vi "CANbus Wrapper.vi"(0 "Signals IN":T4[](array[typedef])=[{"XNET Signal"="GIP_TestModeFlag\nDatabase", "Data"=0.0}, {"XNET Signal"="StatusLED\nDatabase", "Data"=0.0}, {"XNET Signal"="FaultLED\nDatabase", "Data"=0.0}, {"XNET Signal"="Relay\nDatabase", "Data"=0.0}, {"XNET Signal"="ESP32Comms\nDatabase", "Data"=0.0}], 1 "Method":T5=enum."Write Sigs Session", 2 "JSON signals file":path, 3 "DBC File":path, 5 "Frames IN":T1[](array[typedef]) {"Raw Frame"."payload" format="%x"; "Raw Frame"."timestamp" format="%<%.7X\n%x>T"; "Raw Frame"."type" items=["CAN Data"=0, "CAN Remote"=1, "CAN Bus Error"=2, "CAN 2.0 Data"=8, "CAN FD Data"=16, "CAN FD+BRS Data"=24, "J1939 Data"=192, "Delay"=224, "Log Trigger"=225, "Start Trigger"=226]; "Raw Frame"."identifier" format="%x"}, 7 "Baud Rate":u64=1000000, 9 "Termination":u32(ring) items=["Off", "On"], 11 "error in (no error)":errorcluster, 12 "interface":refnum<k21>="CAN2") -> (4 "Signals OUT":T4[](array[typedef]), 6 "Frames OUT":T1[](array[typedef]) {"Raw Frame"."payload" format="%x"; "Raw Frame"."timestamp" format="%<%.7X\n%x>T"; "Raw Frame"."type" items=["CAN Data"=0, "CAN Remote"=1, "CAN Bus Error"=2, "CAN 2.0 Data"=8, "CAN FD Data"=16, "CAN FD+BRS Data"=24, "J1939 Data"=192, "Delay"=224, "Log Trigger"=225, "Start Trigger"=226]; "Raw Frame"."identifier" format="%x"}, 15 "error out":errorcluster)   [LabVIEW 2021]
uses:
  controls/BCS Manager.ctl
  controls/Signal Data.ctl
  controls/Frame Data.ctl
  <vilib>/xnet/xnet.llb/XNET Frame CAN.ctl
  <vilib>/xnet/xnet.llb/XNET Frame Type CAN.ctl
  controls/Signal Tracker.ctl
  <vilib>/xnet/xnet.llb/XNET Create Session (Frame Input Single-point).vi
  <vilib>/xnet/xnet.llb/XNET Create Session (Frame Output Single-point).vi
  <vilib>/xnet/xnet.llb/XNET Create Session (Signal Input Single-point).vi
  <vilib>/xnet/xnet.llb/XNET Create Session (Signal Output Single-point).vi
  <vilib>/xnet/xnet.llb/XNET Write (Signal Single-point).vi
  <vilib>/xnet/xnet.llb/XNET Create Session (Conversion).vi
  <vilib>/xnet/xnet.llb/XNET Convert (Signal to Frame CAN).vi
  <vilib>/xnet/xnet.llb/XNET Write (Frame CAN).vi
  <vilib>/xnet/xnet.llb/XNET Read (Signal Single-point).vi
  <vilib>/xnet/xnet.llb/XNET Read (Frame CAN).vi
  <resource>/objmgr/xnet.rc
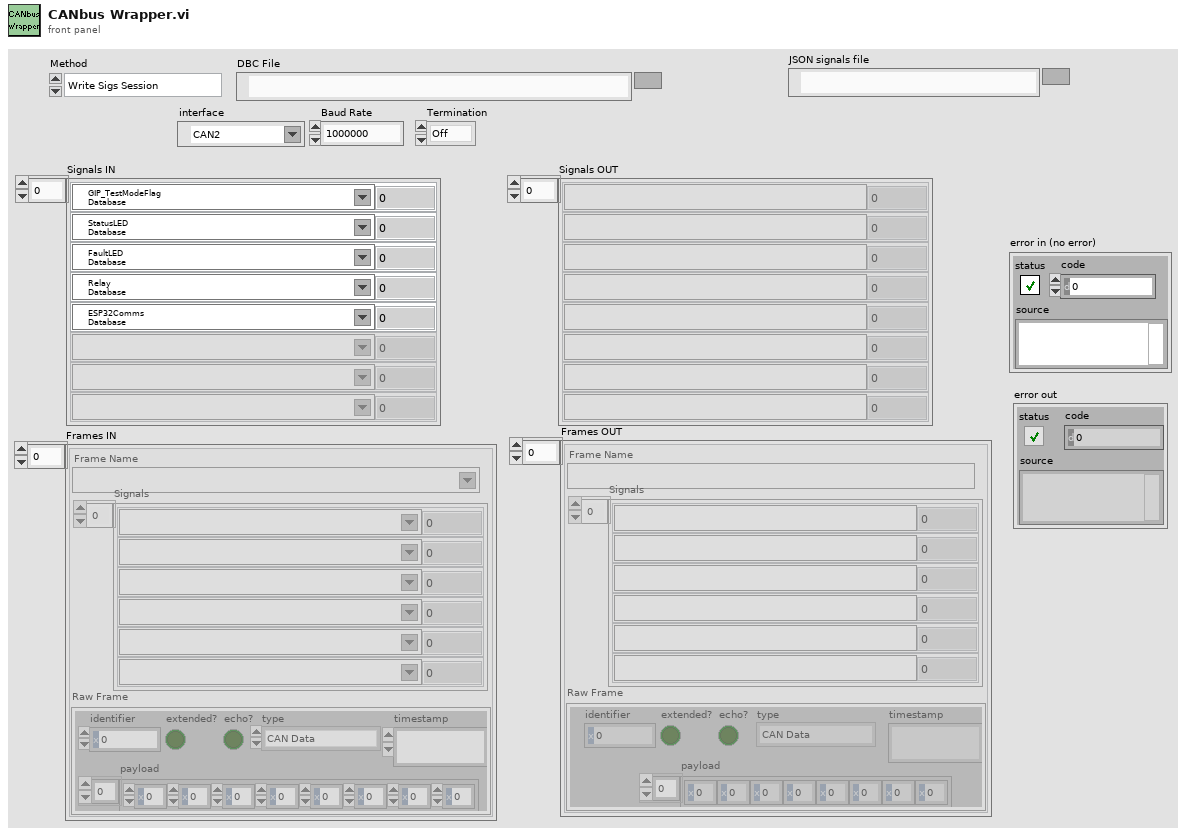
[diagram p1: front panel]
types:
  T1 = typedef "Frame Data.ctl" = cluster{"Raw Frame":T2, "Frame Name":refnum<k21>, "Signals":T4[]}
  T2 = typedef "XNET Frame CAN.ctl" = cluster{"timestamp":timestamp, "payload":u8[], "identifier":u32, "type":T3, "extended?":bool, "echo?":bool}
  T3 = typedef "XNET Frame Type CAN.ctl" = u8
  T4 = typedef "Signal Data.ctl" = cluster{"XNET Signal":refnum<k21>, "Data":dbl}
  T5 = typedef "BCS Manager.ctl" = enum16{"Init", "Start Signal Session", "Start Frame Session", "Write Sigs Session", "Write Frames Session", "Write Sigs Single", "Write Frames Single", "Read Sigs Session", "Read Frames Session", "Read Sigs Single", "Read Frames Single", "Write Raw Frame Session", "Write Raw Frame Single", "FrameRef to Sigs", "FrameID to FrameRef", "Close"}
  T6 = typedef "Signal Tracker.ctl" = enum16{"Init", "Update", "Read", "Clear"}
  T7 = typedef "JSON sigs.ctl" = cluster{"Read Signals Cyclic":refnum<k21>[], "Write Signals Cyclic":refnum<k21>[], "Write Frames Cyclic":refnum<k21>[], "Read Frames Cyclic":refnum<k21>[]}
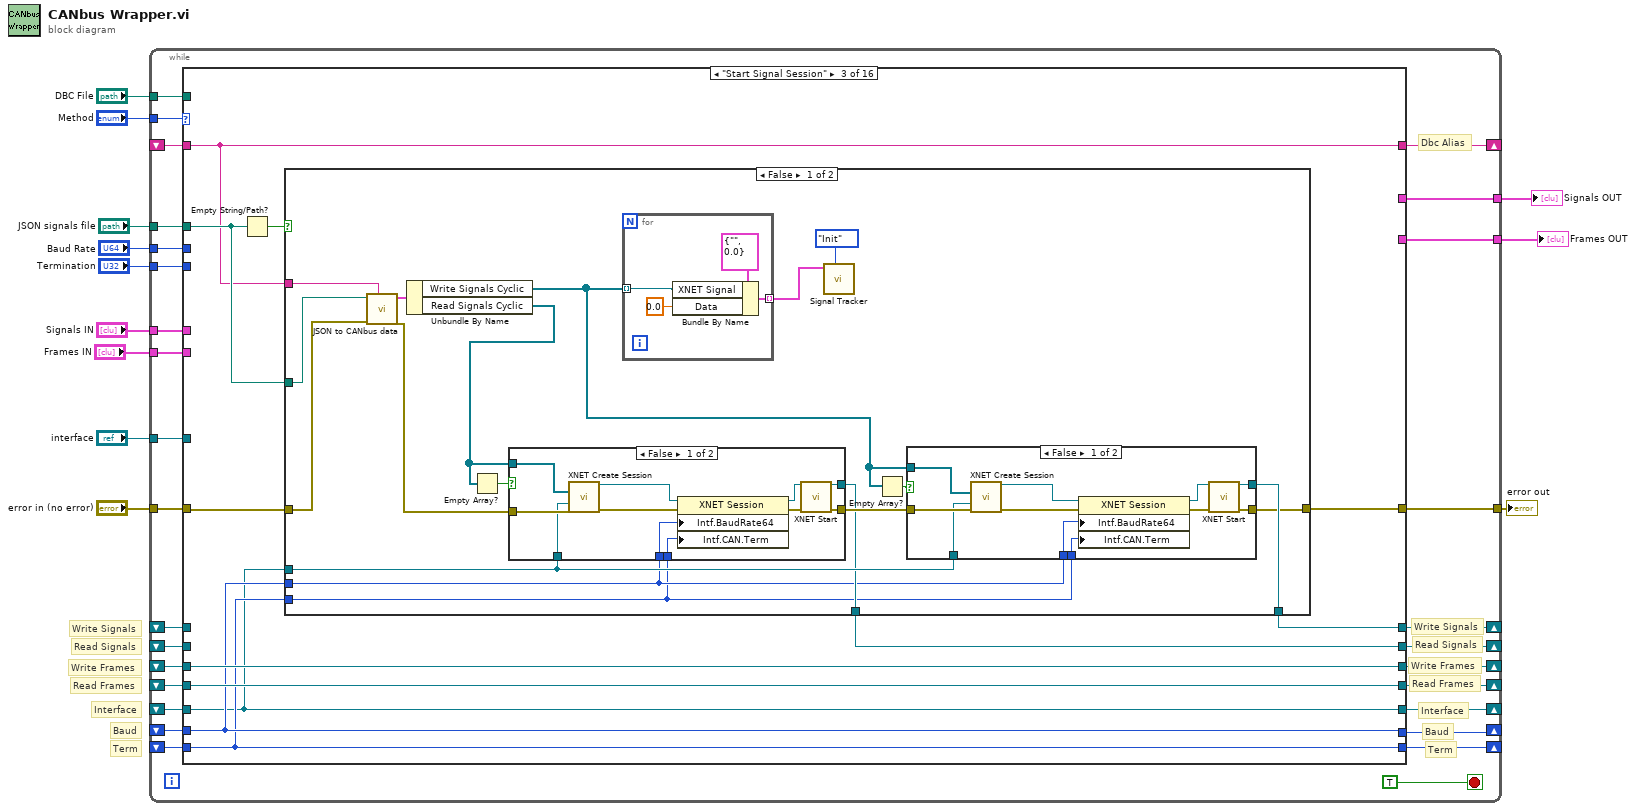
[diagram p0: block diagram]
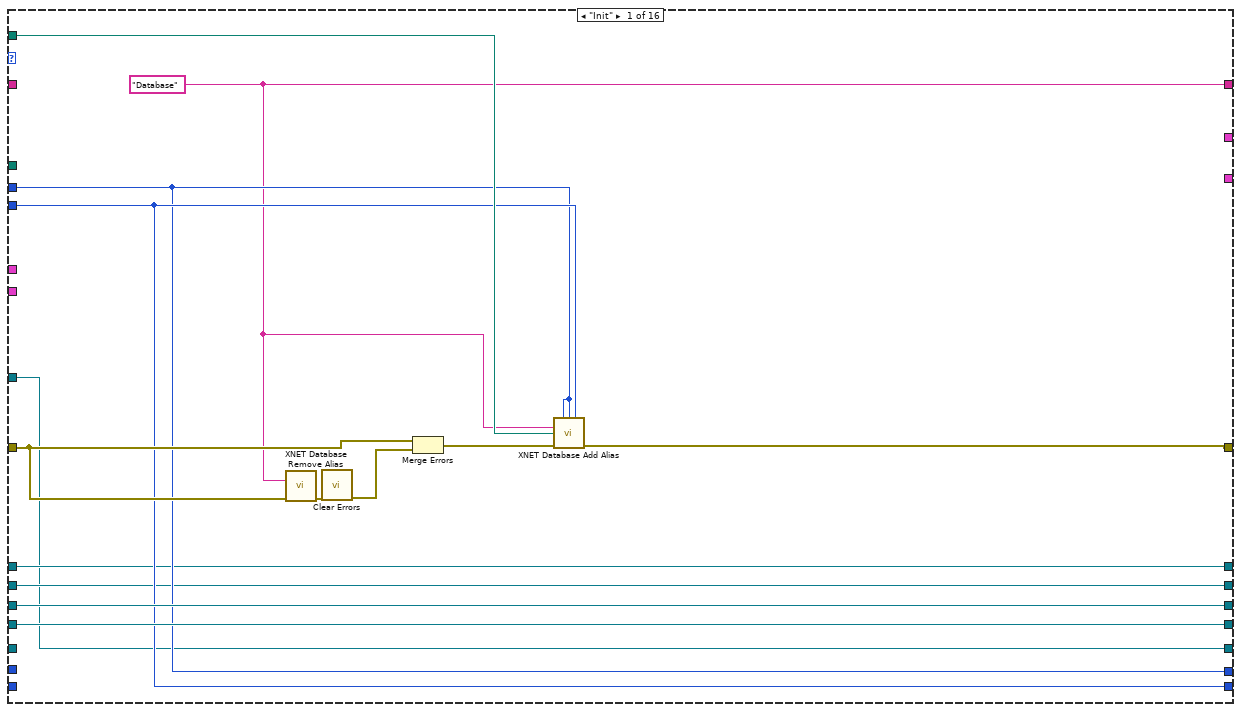
[diagram p2: hidden frame]
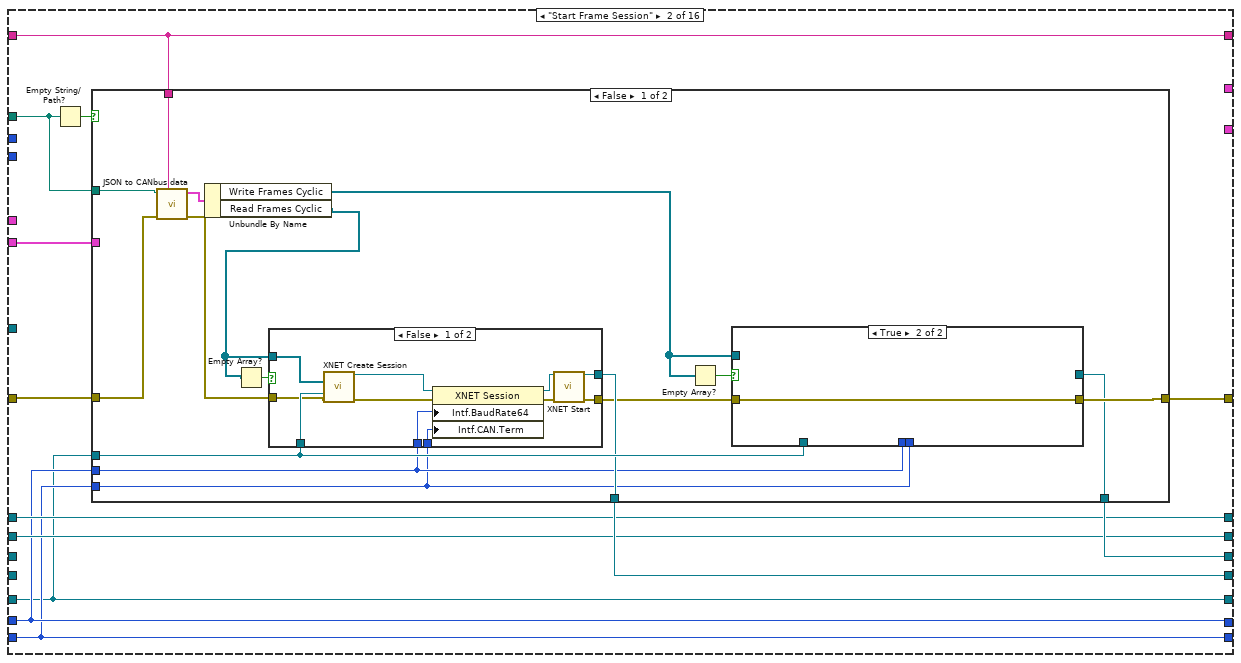
[diagram p3: hidden frame]
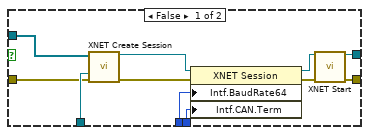
[diagram p4: hidden frame]
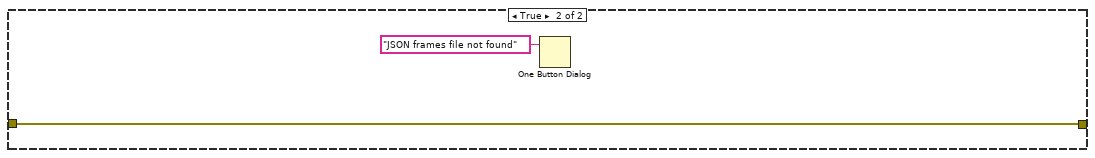
[diagram p6: hidden frame]
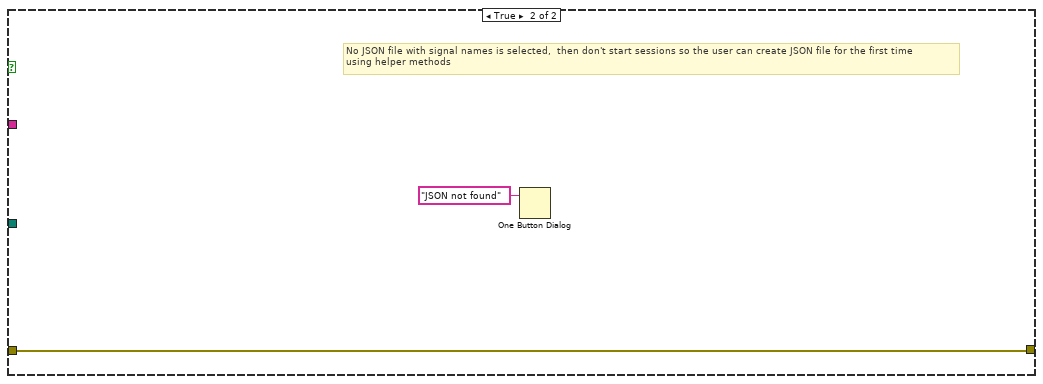
[diagram p9: hidden frame]
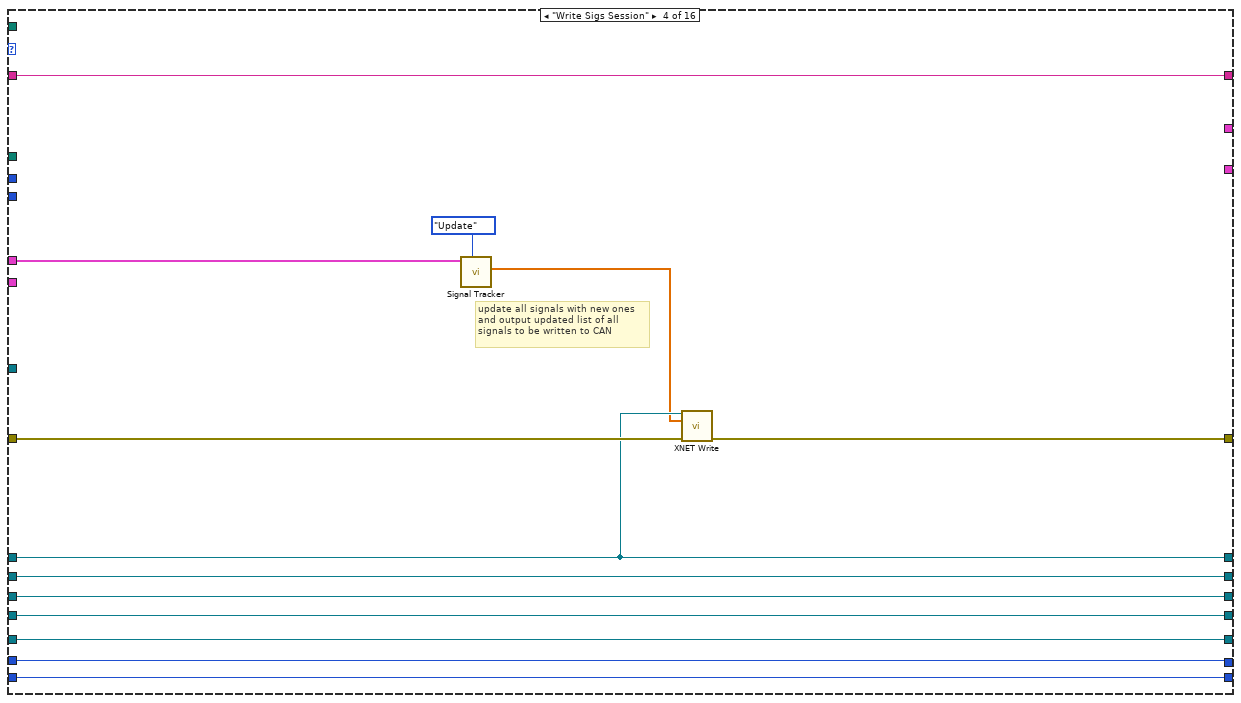
[diagram p10: hidden frame]
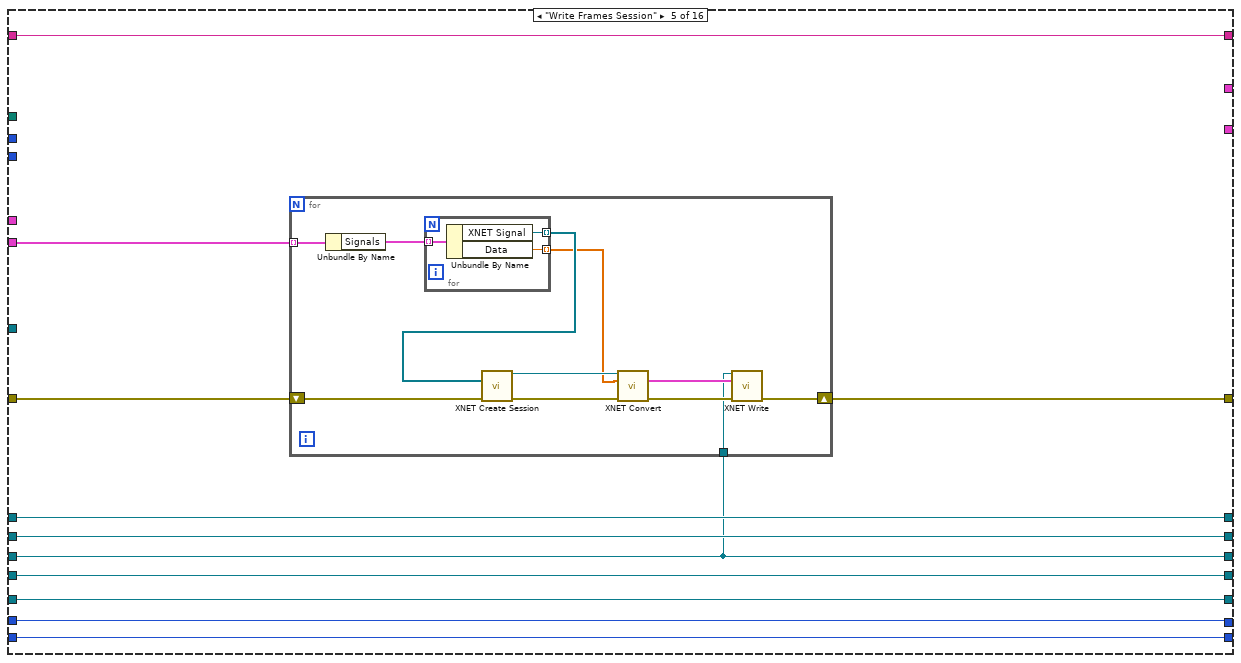
[diagram p11: hidden frame]
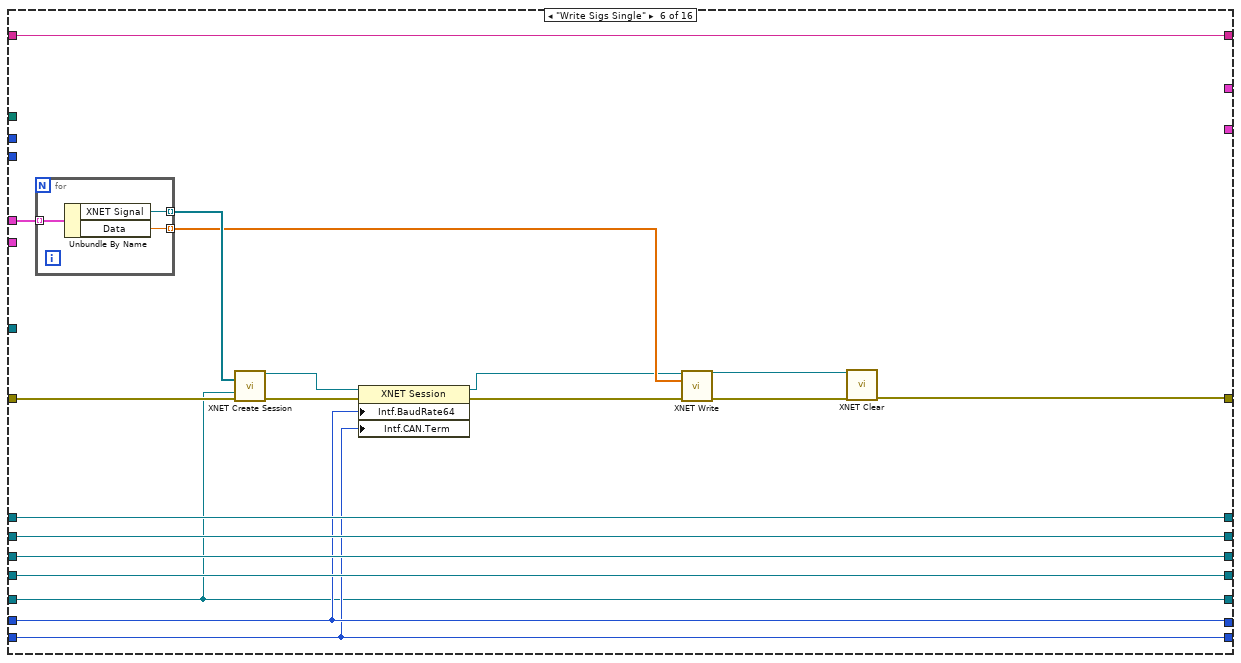
[diagram p12: hidden frame]
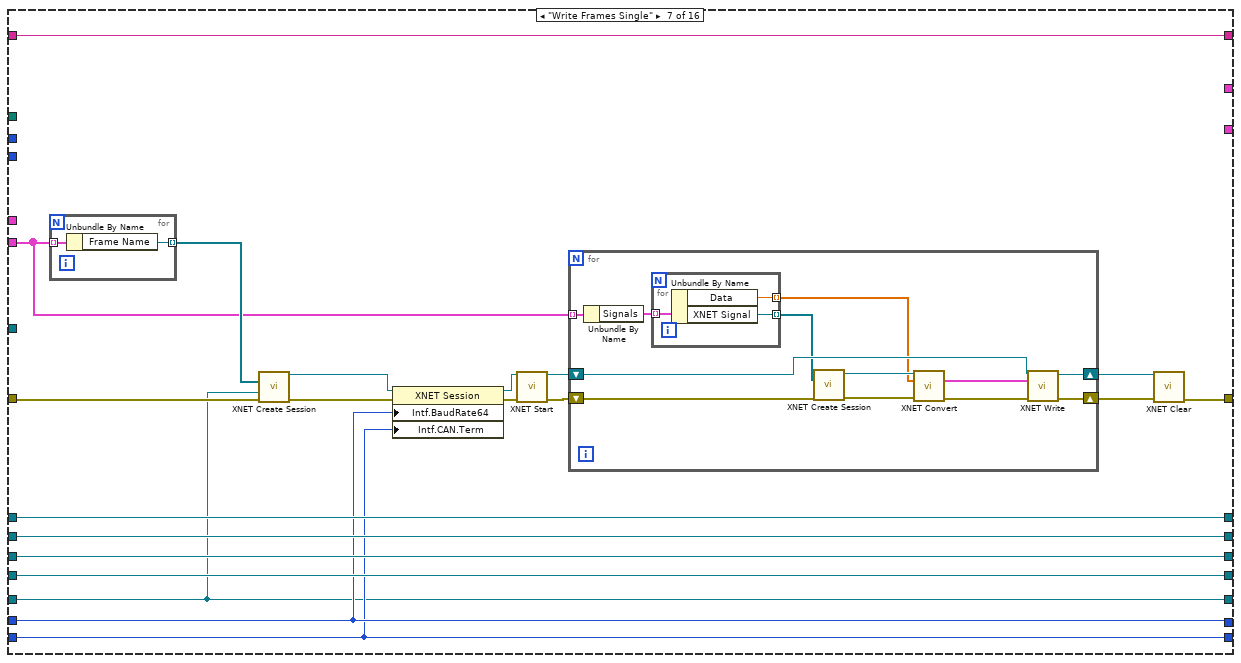
[diagram p13: hidden frame]
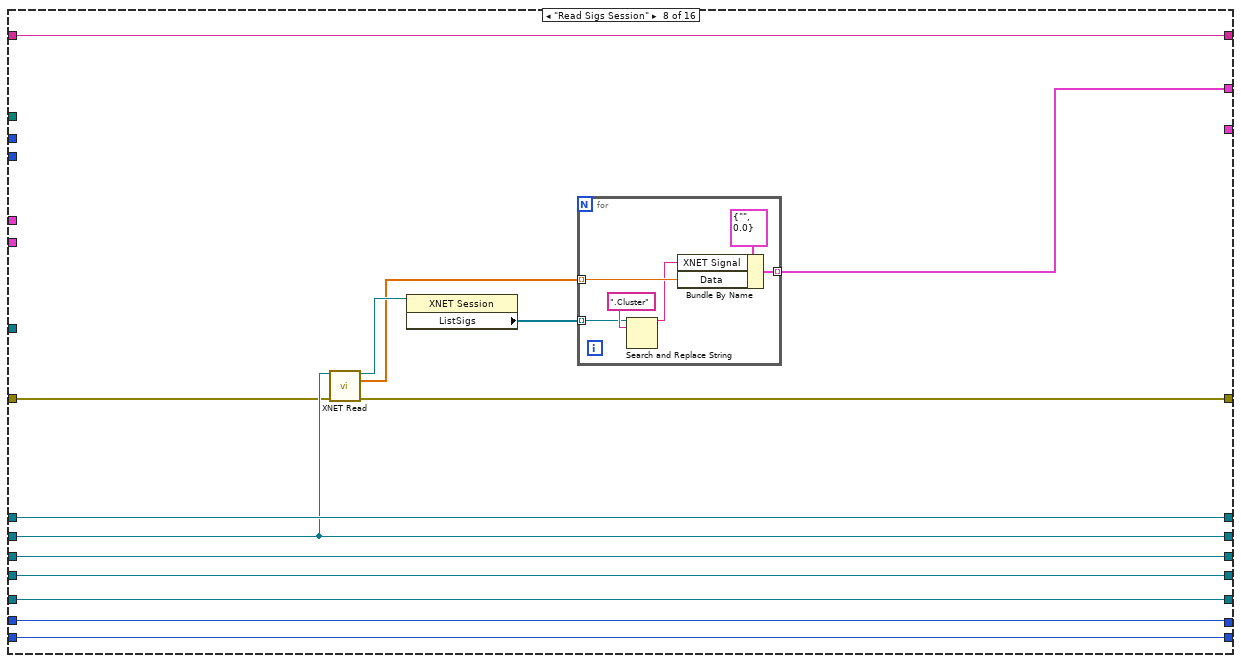
[diagram p14: hidden frame]
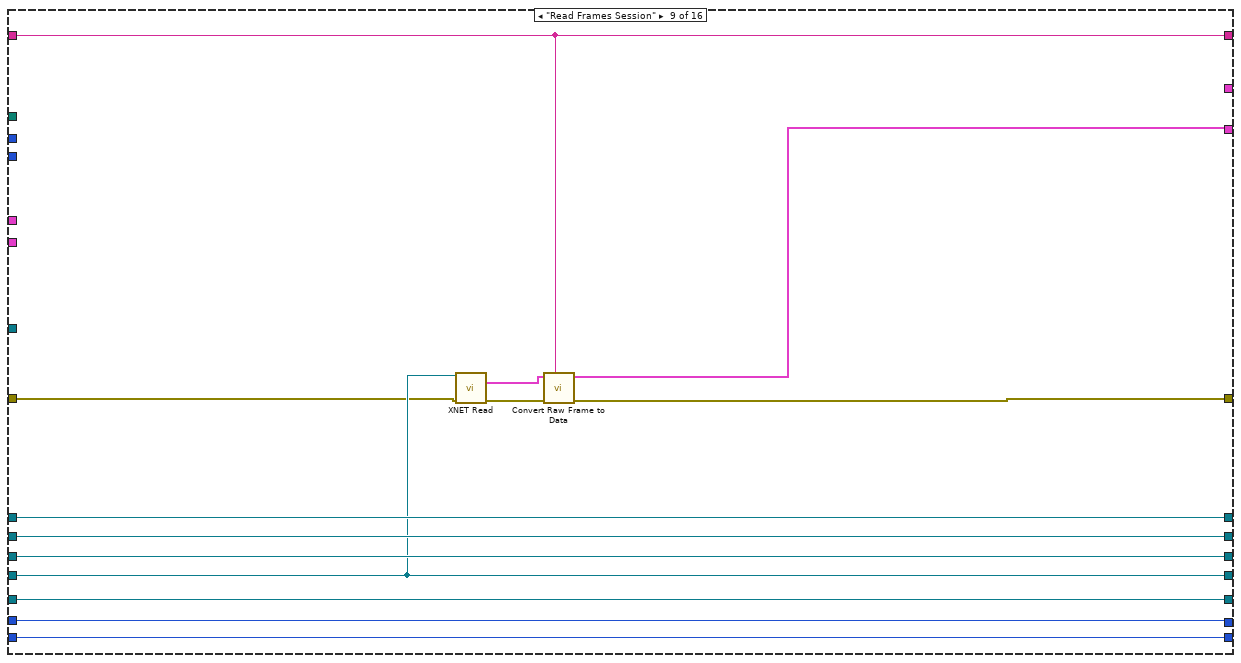
[diagram p15: hidden frame]
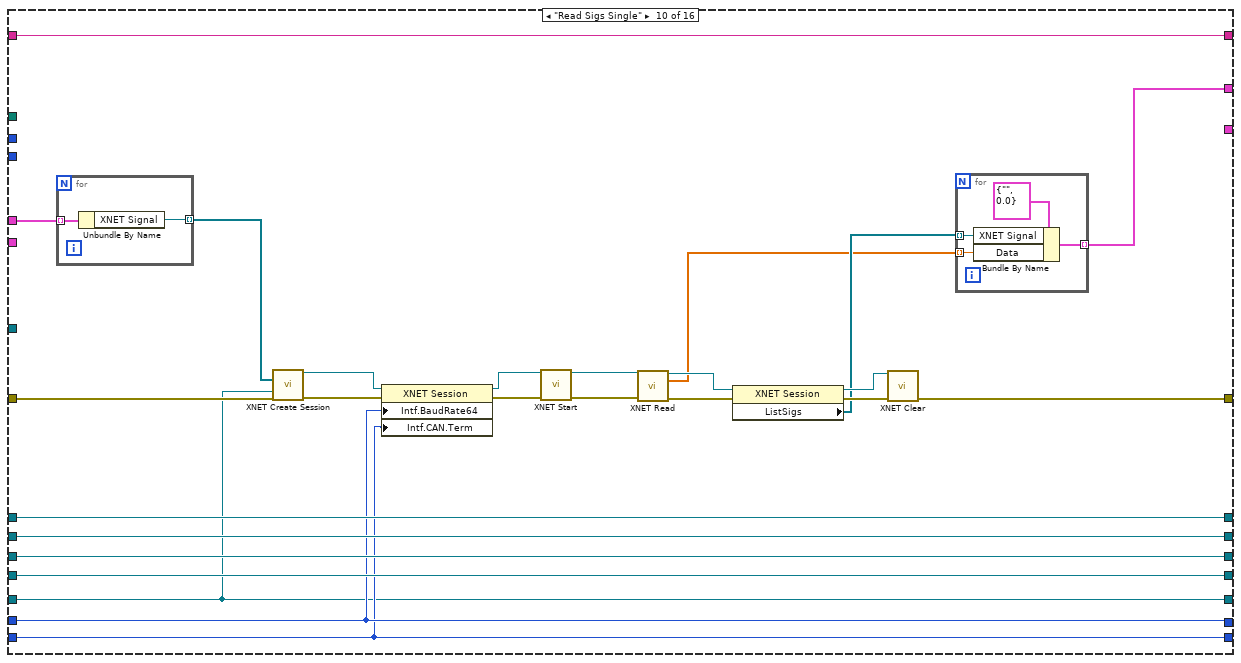
[diagram p16: hidden frame]
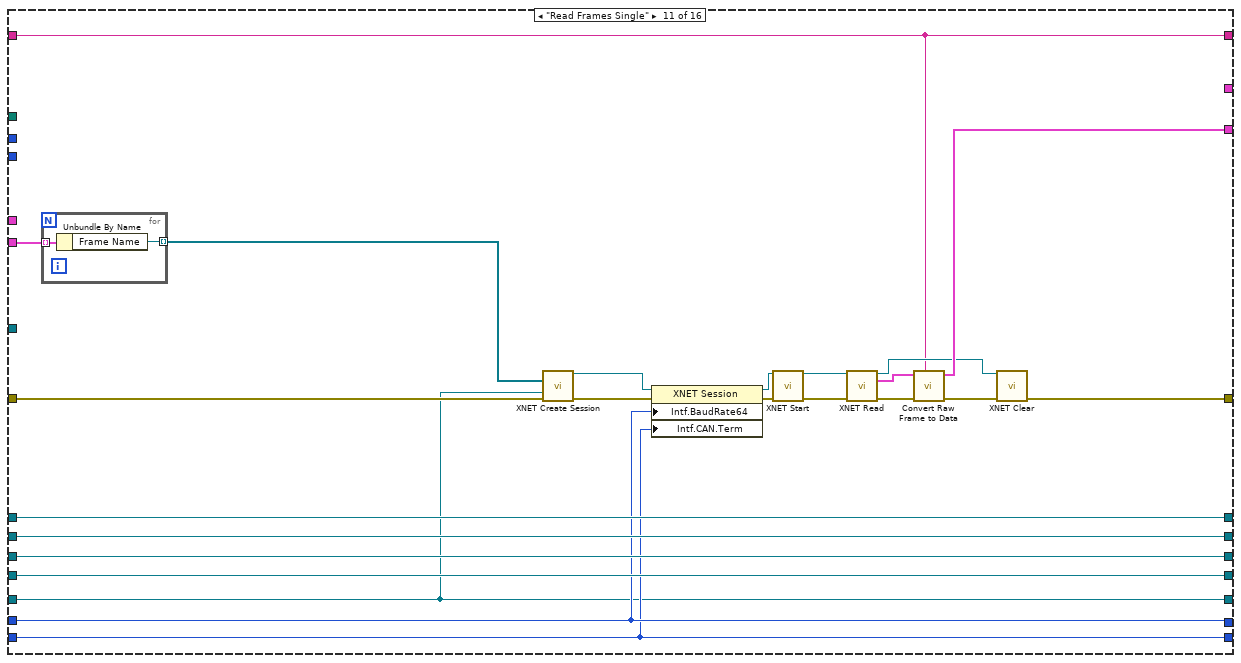
[diagram p17: hidden frame]
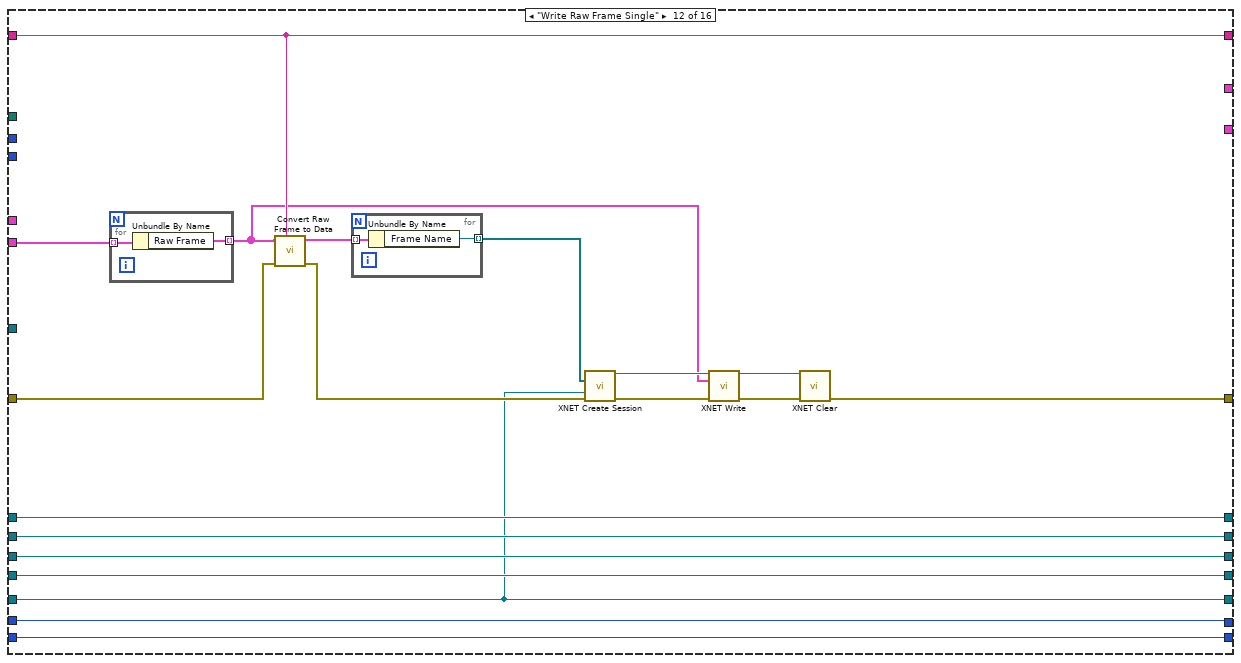
[diagram p18: hidden frame]
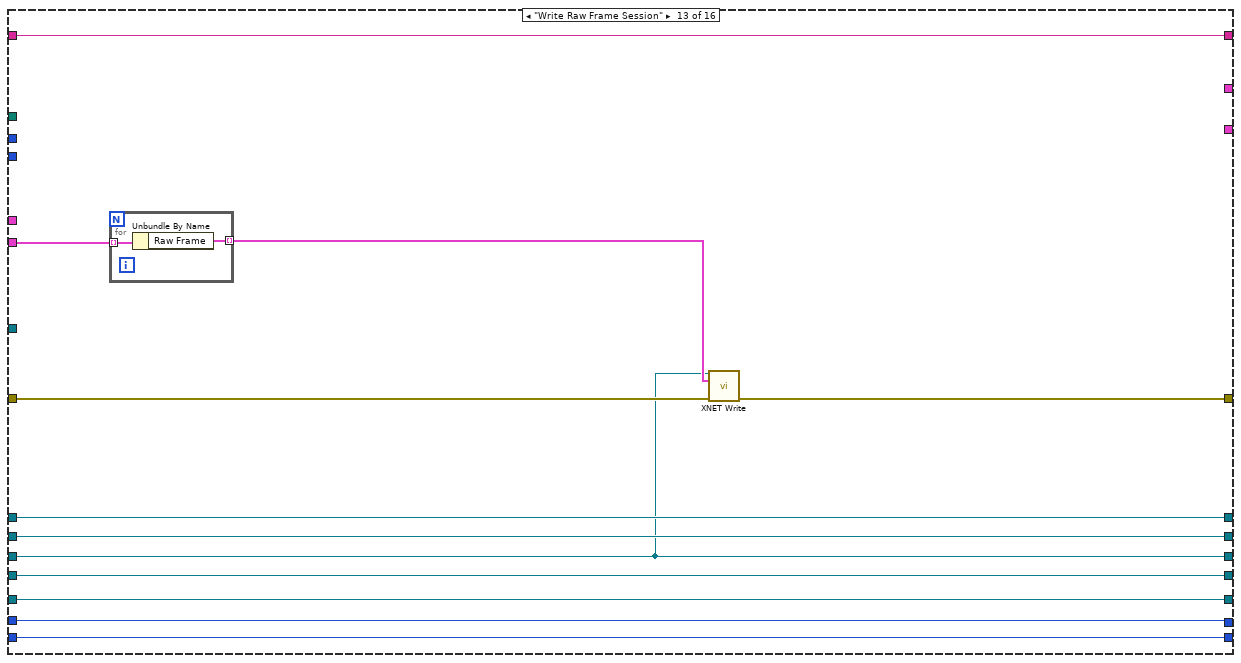
[diagram p19: hidden frame]
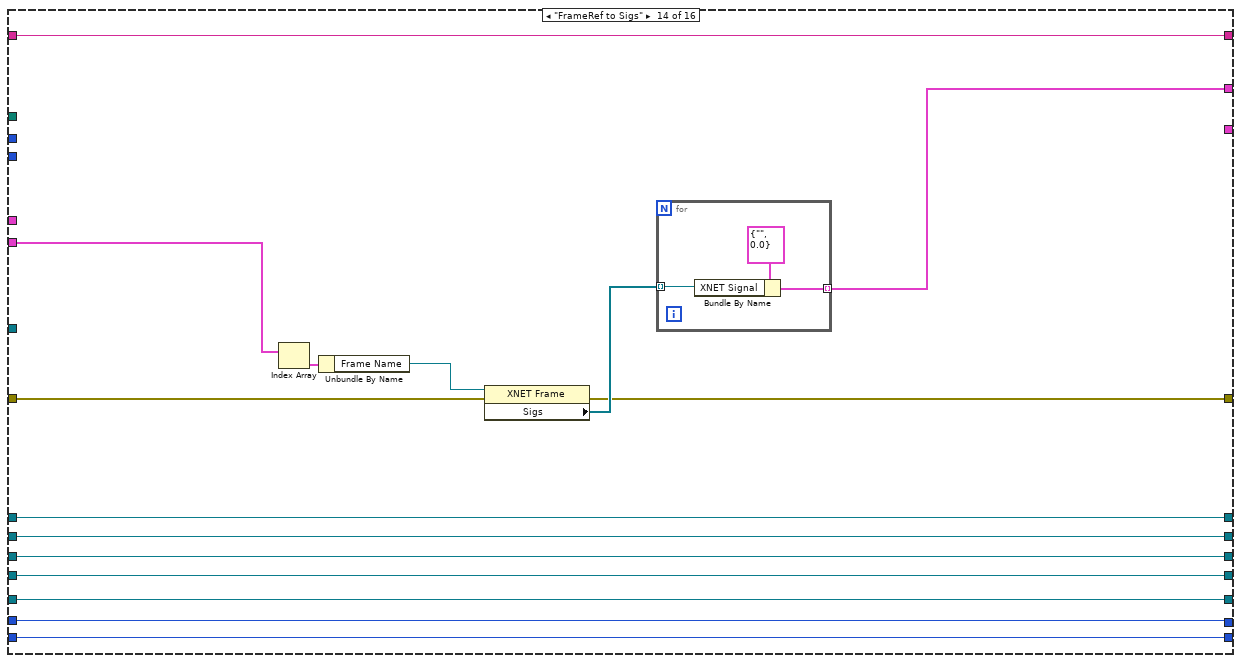
[diagram p20: hidden frame]
diagram:
  # "Interface"
  # "Term"
  # "Baud"
  # "Write Frames"
  # "Read Frames"
  # "Write Signals"
  # "Read Signals"
  n1 = while {
    tunnel: "Method" -> [w40]
    tunnel: "error in (no error)" -> [w39]
    tunnel: "DBC File" -> [w38]
    tunnel: [w37] -> w9
    tunnel: "interface" -> [w36]
    tunnel: "Signals IN" -> [w35]
    shift-right: [w34] -> _
    shift-left: _ -> [w33]
    tunnel: "JSON signals file" -> [w32]
    shift-right: [w30] -> _
    shift-left: _ -> [w31]
    tunnel: "Frames IN" -> [w29]
    tunnel: [w28] -> w4
    tunnel: [w27] -> w3
    shift-right: [w23] -> _
    shift-left: _ -> [w24]
    shift-right: [w26] -> _
    shift-left: _ -> [w25]
    shift-right: [w19] -> _
    shift-left: _ -> [w18]
    shift-right: [w20] -> _
    shift-left: _ -> [w17]
    tunnel: "Baud Rate" -> [w22]
    tunnel: "Termination" -> [w21]
    shift-right: [w16] -> _
    shift-left: _ -> [w15]
    shift-right: [w14] -> _
    shift-left: _ -> [w13]
    stop <- TRUE stop-if-true
    # "Interface"
    # "Dbc Alias"
    # "Term"
    # "Baud"
    # "Write Frames"
    # "Read Frames"
    # "Write Signals"
    # "Read Signals"
    n2 = case shown="\"Start Signal Session\"" w40 {
      tunnel: w39 -> [w49 w65 w117 w182 w193 w223 w244 w278 w288 w319 w341 w360 w383 w400 w415 w440]
      tunnel: w38 -> [w55 _ _ _ _ _ _ _ _ _ _ _ _ _ _ _]
      tunnel: [w42 w68 w122 w181 w192 w220 w240 w281 w300 w316 w339 w370 w381 w397 w414 w427] -> w37
      tunnel: w36 -> [w44 _ _ _ _ _ _ _ _ _ _ _ _ _ _ _]
      tunnel: w35 -> [_ _ _ w172 _ w217 _ _ _ w311 _ _ _ _ _ _]
      tunnel: [w45 w61 w121 w183 w194 w227 w250 w279 w296 w324 w353 w373 w391 w408 w425 w435] -> w34
      tunnel: w33 -> [w45 w61 _ w183 w194 w227 w250 w279 w296 w324 w353 w373 w391 w408 w425 w435]
      tunnel: w32 -> [_ w66 w119 _ _ _ _ _ _ _ _ _ _ _ _ _]
      tunnel: [w46 w62 w120 w180 w191 w226 w249 w280 w299 w325 w354 w369 w390 w407 w424 w436] -> w30
      tunnel: w31 -> [w46 w62 _ w180 w191 w226 w249 w280 w299 w325 w354 w369 w390 w407 w424 w436]
      tunnel: w29 -> [_ w57 _ _ w186 _ w235 _ _ _ w344 w364 w386 w401 w419 _]
      tunnel: [_ _ _ _ _ _ _ _ w293 _ w342 _ _ _ _ _] -> w28
      tunnel: [_ _ _ _ _ _ _ w274 _ w307 _ _ _ w398 _ _] -> w27
      tunnel: [w51 w63 w116 w177 w190 w218 w237 w272 w294 w305 w336 w367 w389 w405 w422 w433] -> w23
      tunnel: w24 -> [w51 _ w116 w177 w190 w218 w237 w272 w294 w305 w336 w367 w389 w405 w422 w433]
      tunnel: [w52 w64 w115 w178 w189 w219 w238 w273 w295 w306 w337 w368 w382 w406 w423 w434] -> w26
      tunnel: w25 -> [w52 _ w115 w178 w189 w219 w238 w273 w295 w306 w337 w368 w382 w406 w423 w434]
      tunnel: w22 -> [w47 _ _ _ _ _ _ _ _ _ _ _ _ _ _ _]
      tunnel: w21 -> [w48 _ _ _ _ _ _ _ _ _ _ _ _ _ _ _]
      tunnel: [w48 w59 w113 w175 w187 w213 w233 w270 w291 w303 w334 w365 w387 w403 w420 w438] -> w20
      tunnel: [w47 w60 w114 w176 w188 w214 w234 w271 w292 w304 w335 w366 w388 w404 w421 w439] -> w19
      tunnel: w18 -> [_ w60 w114 w176 w188 w214 w234 w271 w292 w304 w335 w366 w388 w404 w421 w439]
      tunnel: w17 -> [_ w59 w113 w175 w187 w213 w233 w270 w291 w303 w334 w365 w387 w403 w420 w438]
      tunnel: [w43 w58 w112 w174 w185 w212 w232 w269 w290 w302 w333 w363 w385 w402 w413 w426] -> w16
      tunnel: w15 -> [_ w58 w112 w174 w185 w212 w232 w269 w290 w302 w333 w363 w385 w402 w413 w426]
      tunnel: [w44 w56 w111 w173 w184 w211 w231 w268 w289 w301 w332 w357 w380 w396 w412 w437] -> w14
      tunnel: w13 -> [_ w56 w111 w173 w184 w211 w231 w268 w289 w301 w332 w357 w380 w396 w412 w437]
      frame "Init" {
        w43 = "Database"
        n3 = call <vilib>:"XNET Database Remove Alias.vi"("alias"=w43, "error in (no error)"=w49) -> ("error out"=w54:errorcluster)  [unwired: 13 in]
        n4 = call <vilib>:"Clear Errors.vi"("error in (no error)"=w54) -> ("error out"=w53:errorcluster)  [unwired: 5 in, 1 out]
        n5 = Merge Errors(w49, w53) -> (w50:errorcluster)
        n6 = call <vilib>:"XNET Database Add Alias.vi"("default baud rate (0)"=w47, "default FD baud rate (0)"=w47, "CAN FD ISO mode (ISO)"=w48, "alias"=w43, "filepath"=w55, "error in (no error)"=w50) -> ("error out"=w42:errorcluster)  [unwired: 9 in]
      }
      frame "Start Frame Session" {
        n7 = Empty String/Path?(string/path=w66) -> (empty?=w67:bool)
        n8 = case shown="False" w67 {
          tunnel: w56 -> [w84 _]
          tunnel: [w83 w109] -> w68
          tunnel: [w82 _] -> w63
          tunnel: [w81 _] -> w64
          tunnel: w58 -> [w72 _]
          tunnel: w66 -> [w71 _]
          tunnel: w65 -> [w69 w109]
          tunnel: w60 -> [w79 _]
          tunnel: w59 -> [w78 _]
          tunnel: w57 -> [_ _]
          frame False {
            n9 = call "JSON to CANbus data.vi"("Database Alias"=w72, "error in"=w69, "JSON file"=w71) -> ("error out"=w70:errorcluster, "Signal Sessions"=w77:T7)  [unwired: 7 in]
            n10 = Unbundle By Name(w77) -> ("Write Frames Cyclic"=w73:refnum<k21>[], "Read Frames Cyclic"=w75:refnum<k21>[])
            n11 = Empty Array?(array=w75) -> (empty?=w76:bool)
            n12 = case shown="False" w76 {
              tunnel: w84 -> [w107 _]
              tunnel: [w106 _] -> w82
              tunnel: [w105 w108] -> w80
              tunnel: w70 -> [w100 w108]
              tunnel: w79 -> [w99 _]
              tunnel: w78 -> [w98 _]
              tunnel: w75 -> [w97 _]
              frame False {
                n13 = call-poly <vilib>:"XNET Create Session.vi"("frame list"=w97, "interface"=w107, "error in (no error)"=w100) -> ("session out"=w102:refnum<k21>, "error out"=w104:errorcluster)  [unwired: 11 in]
                n14 = property class="XNET Session"(reference=w102, error in=w104, "Intf.BaudRate64"=w99, "Intf.CAN.Term"=w98) -> (reference out=w101:refnum<k21>, error out=w103:errorcluster)
                n15 = call <vilib>:"XNET Start.vi"("session in"=w101, "error in (no error)"=w103) -> ("session out"=w106:refnum<k21>, "error out"=w105:errorcluster)  [unwired: 12 in]
              }
              frame True {
              }
            }
            n16 = Empty Array?(array=w73) -> (empty?=w74:bool)
            n17 = case shown="True" w74 {
              tunnel: w84 -> [w95 _]
              tunnel: [w94 w96] -> w83
              tunnel: [w93 _] -> w81
              tunnel: w80 -> [w88 w96]
              tunnel: w79 -> [w87 _]
              tunnel: w78 -> [w86 _]
              tunnel: w73 -> [w85 _]
              frame False {
                n18 = call-poly <vilib>:"XNET Create Session.vi"("frame list"=w85, "interface"=w95, "error in (no error)"=w88) -> ("session out"=w92:refnum<k21>, "error out"=w90:errorcluster)  [unwired: 11 in]
                n19 = property class="XNET Session"(reference=w92, error in=w90, "Intf.BaudRate64"=w87, "Intf.CAN.Term"=w86) -> (reference out=w91:refnum<k21>, error out=w89:errorcluster)
                n20 = call <vilib>:"XNET Start.vi"("session in"=w91, "error in (no error)"=w89) -> ("session out"=w93:refnum<k21>, "error out"=w94:errorcluster)  [unwired: 12 in]
              }
              frame True {
              }
            }
          }
          frame True {
            n21 = One Button Dialog(message="JSON frames file not found") -> ()  [unwired: 1 in, 1 out]
          }
        }
      }
      frame "Start Signal Session" {
        n22 = Empty String/Path?(string/path=w119) -> (empty?=w118:bool)
        n23 = case shown="False" w118 {
          tunnel: w111 -> [w138 _]
          tunnel: [w137 _] -> w121
          tunnel: w112 -> [w135 _]
          tunnel: [w130 w170] -> w122
          tunnel: [w131 _] -> w120
          tunnel: w119 -> [w124 _]
          tunnel: w117 -> [w123 w170]
          tunnel: w114 -> [w133 _]
          tunnel: w113 -> [w132 _]
          frame False {
            n24 = call "JSON to CANbus data.vi"("Database Alias"=w135, "error in"=w123, "JSON file"=w124) -> ("error out"=w139:errorcluster, "Signal Sessions"=w134:T7)  [unwired: 7 in]
            n25 = Unbundle By Name(w134) -> ("Write Signals Cyclic"=w126:refnum<k21>[], "Read Signals Cyclic"=w127:refnum<k21>[])
            n26 = Empty Array?(array=w127) -> (empty?=w129:bool)
            n27 = case shown="False" w129 {
              tunnel: [w163 w168] -> w140
              tunnel: w139 -> [w162 w168]
              tunnel: w138 -> [w161 _]
              tunnel: [w160 _] -> w137
              tunnel: w133 -> [w159 _]
              tunnel: w132 -> [w158 _]
              tunnel: w127 -> [w157 _]
              frame False {
                n28 = call-poly <vilib>:"XNET Create Session.vi"("signal list"=w157, "interface"=w161, "error in (no error)"=w162) -> ("session out"=w164:refnum<k21>, "error out"=w166:errorcluster)  [unwired: 11 in]
                n29 = property class="XNET Session"(reference=w164, error in=w166, "Intf.BaudRate64"=w159, "Intf.CAN.Term"=w158) -> (reference out=w165:refnum<k21>, error out=w167:errorcluster)
                n30 = call <vilib>:"XNET Start.vi"("session in"=w165, "error in (no error)"=w167) -> ("session out"=w160:refnum<k21>, "error out"=w163:errorcluster)  [unwired: 12 in]
              }
              frame True {
              }
            }
            n31 = for {
              tunnel: w126 -> [w142] mode=indexing
              tunnel: [w141] -> w125 mode=indexing
              n32 = Bundle By Name(cluster=T4 {"XNET Signal"="", "Data"=0.0} ("Signals IN"), "XNET Signal"=w142, "Data"=0.0) -> (w141:T4)
            }
            n33 = call "Signal Tracker.vi"("Action"=Signal_Tracker."Init", "Signals"=w125) -> ()  [unwired: 7 in, 3 out]
            n34 = Empty Array?(array=w126) -> (empty?=w128:bool)
            n35 = case shown="False" w128 {
              tunnel: w140 -> [w151 w156]
              tunnel: w138 -> [w150 _]
              tunnel: w133 -> [w149 _]
              tunnel: w132 -> [w148 _]
              tunnel: [w147 _] -> w131
              tunnel: [w146 w156] -> w130
              tunnel: w126 -> [w145 _]
              frame False {
                n36 = call-poly <vilib>:"XNET Create Session.vi"("signal list"=w145, "interface"=w150, "error in (no error)"=w151) -> ("session out"=w155:refnum<k21>, "error out"=w153:errorcluster)  [unwired: 11 in]
                n37 = property class="XNET Session"(reference=w155, error in=w153, "Intf.BaudRate64"=w149, "Intf.CAN.Term"=w148) -> (reference out=w154:refnum<k21>, error out=w152:errorcluster)
                n38 = call <vilib>:"XNET Start.vi"("session in"=w154, "error in (no error)"=w152) -> ("session out"=w147:refnum<k21>, "error out"=w146:errorcluster)  [unwired: 12 in]
              }
              frame True {
              }
            }
          }
          frame True {
            # "No JSON file with signal names is selected,  then don't start sessions so the user can create JSON file for the first time\nusing helper methods"
            n39 = One Button Dialog(message="JSON not found") -> ()  [unwired: 1 in, 1 out]
          }
        }
      }
      frame "Write Sigs Session" {
        # "update all signals with new ones\nand output updated list of all\nsignals to be written to CAN"
        n40 = call "Signal Tracker.vi"("Action"=Signal_Tracker."Update", "Signals"=w172) -> ("Signal Values"=w171:dbl[])  [unwired: 7 in, 2 out]
        n41 = call-poly <vilib>:"XNET Write.vi"("session in"=w180, "data"=w171, "error in (no error)"=w182) -> ("error out"=w181:errorcluster)  [unwired: 11 in, 1 out]
      }
      frame "Write Frames Session" {
        n42 = for {
          tunnel: w189 -> [w199]
          shift-right: [w204] -> w192
          shift-left: w193 -> [w205]
          tunnel: w186 -> [w198] mode=indexing
          n43 = Unbundle By Name(w198) -> ("Signals"=w197:T4[])
          n44 = for {
            tunnel: w197 -> [w208] mode=indexing
            tunnel: [w207] -> w196 mode=indexing
            tunnel: [w206] -> w195 mode=indexing
            n45 = Unbundle By Name(w208) -> ("XNET Signal"=w207:refnum<k21>, "Data"=w206:dbl)
          }
          n46 = call-poly <vilib>:"XNET Create Session.vi"("signal list"=w196, "error in (no error)"=w205) -> ("session out"=w202:refnum<k21>, "error out"=w203:errorcluster)  [unwired: 12 in]
          n47 = call-poly <vilib>:"XNET Convert.vi"("session in"=w202, "signal data"=w195, "error in (no error)"=w203) -> ("frame data"=w201:T2[], "error out"=w200:errorcluster)  [unwired: 9 in, 2 out]
          n48 = call-poly <vilib>:"XNET Write.vi"("session in"=w199, "data"=w201, "error in (no error)"=w200) -> ("error out"=w204:errorcluster)  [unwired: 11 in, 1 out]
        }
      }
      frame "Write Sigs Single" {
        n49 = for {
          tunnel: w217 -> [w230] mode=indexing
          tunnel: [w229] -> w216 mode=indexing
          tunnel: [w228] -> w215 mode=indexing
          n50 = Unbundle By Name(w230) -> ("XNET Signal"=w229:refnum<k21>, "Data"=w228:dbl)
        }
        n51 = call-poly <vilib>:"XNET Create Session.vi"("signal list"=w216, "interface"=w211, "error in (no error)"=w223) -> ("session out"=w225:refnum<k21>, "error out"=w224:errorcluster)  [unwired: 11 in]
        n52 = property class="XNET Session"(reference=w225, error in=w224, "Intf.BaudRate64"=w214, "Intf.CAN.Term"=w213) -> (reference out=w210:refnum<k21>, error out=w209:errorcluster)
        n53 = call-poly <vilib>:"XNET Write.vi"("session in"=w210, "data"=w215, "error in (no error)"=w209) -> ("session out"=w221:refnum<k21>, "error out"=w222:errorcluster)  [unwired: 11 in]
        n54 = call <vilib>:"XNET Clear.vi"("session in"=w221, "error in (no error)"=w222) -> ("error out"=w220:errorcluster)  [unwired: 13 in]
      }
      frame "Write Frames Single" {
        n55 = for {
          tunnel: w235 -> [w267] mode=indexing
          tunnel: [w266] -> w236 mode=indexing
          n56 = Unbundle By Name(w267) -> ("Frame Name"=w266:refnum<k21>)
        }
        n57 = call-poly <vilib>:"XNET Create Session.vi"("frame list"=w236, "interface"=w231, "error in (no error)"=w244) -> ("session out"=w248:refnum<k21>, "error out"=w246:errorcluster)  [unwired: 11 in]
        n58 = property class="XNET Session"(reference=w248, error in=w246, "Intf.BaudRate64"=w234, "Intf.CAN.Term"=w233) -> (reference out=w247:refnum<k21>, error out=w245:errorcluster)
        n59 = call <vilib>:"XNET Start.vi"("session in"=w247, "error in (no error)"=w245) -> ("session out"=w239:refnum<k21>, "error out"=w243:errorcluster)  [unwired: 12 in]
        n60 = for {
          shift-right: [w257] -> w242
          shift-left: w243 -> [w258]
          shift-right: [w256] -> w241
          shift-left: w239 -> [w255]
          tunnel: w235 -> [w254] mode=indexing
          n61 = Unbundle By Name(w254) -> ("Signals"=w253:T4[])
          n62 = for {
            tunnel: w253 -> [w265] mode=indexing
            tunnel: [w264] -> w252 mode=indexing
            tunnel: [w263] -> w251 mode=indexing
            n63 = Unbundle By Name(w265) -> ("Data"=w264:dbl, "XNET Signal"=w263:refnum<k21>)
          }
          n64 = call-poly <vilib>:"XNET Create Session.vi"("signal list"=w251, "error in (no error)"=w258) -> ("session out"=w261:refnum<k21>, "error out"=w262:errorcluster)  [unwired: 12 in]
          n65 = call-poly <vilib>:"XNET Convert.vi"("session in"=w261, "signal data"=w252, "error in (no error)"=w262) -> ("frame data"=w260:T2[], "error out"=w259:errorcluster)  [unwired: 9 in, 2 out]
          n66 = call-poly <vilib>:"XNET Write.vi"("session in"=w255, "data"=w260, "error in (no error)"=w259) -> ("session out"=w256:refnum<k21>, "error out"=w257:errorcluster)  [unwired: 11 in]
        }
        n67 = call <vilib>:"XNET Clear.vi"("session in"=w241, "error in (no error)"=w242) -> ("error out"=w240:errorcluster)  [unwired: 13 in]
      }
      frame "Read Sigs Session" {
        n68 = call-poly <vilib>:"XNET Read.vi"("session in"=w279, "error in (no error)"=w278) -> ("session out"=w277:refnum<k21>, "data"=w275:dbl[], "error out"=w281:errorcluster)  [unwired: 11 in]
        n69 = property class="XNET Session"(reference=w277) -> ("ListSigs"=w276:refnum<k21>[])  [unwired: 1 in, 2 out]
        n70 = for {
          tunnel: w276 -> [w284] mode=indexing
          tunnel: w275 -> [w285] mode=indexing
          tunnel: [w283] -> w274 mode=indexing
          n71 = Search and Replace String(input string=w284, search string=".Cluster") -> (result string=w282:string)  [unwired: 6 in, 3 out]
          n72 = Bundle By Name(cluster=T4 {"XNET Signal"="", "Data"=0.0} ("Signals OUT"), "XNET Signal"=w282, "Data"=w285) -> (w283:T4)
        }
      }
      frame "Read Frames Session" {
        n73 = call-poly <vilib>:"XNET Read.vi"("session in"=w294, "error in (no error)"=w288) -> ("data"=w297:T2[], "error out"=w298:errorcluster)  [unwired: 10 in, 2 out]
        n74 = call "Convert Raw Frame to Data.vi"("Database alias"=w290, "error in (no error)"=w298, "Raw Frames"=w297) -> ("error out"=w300:errorcluster, "Frame Data"=w293:T1[])  [unwired: 7 in]
      }
      frame "Read Sigs Single" {
        n75 = for {
          tunnel: w311 -> [w331] mode=indexing
          tunnel: [w330] -> w310 mode=indexing
          n76 = Unbundle By Name(w331) -> ("XNET Signal"=w330:refnum<k21>)
        }
        n77 = call-poly <vilib>:"XNET Create Session.vi"("signal list"=w310, "interface"=w301, "error in (no error)"=w319) -> ("session out"=w320:refnum<k21>, "error out"=w322:errorcluster)  [unwired: 11 in]
        n78 = property class="XNET Session"(reference=w320, error in=w322, "Intf.BaudRate64"=w304, "Intf.CAN.Term"=w303) -> (reference out=w321:refnum<k21>, error out=w323:errorcluster)
        n79 = call <vilib>:"XNET Start.vi"("session in"=w321, "error in (no error)"=w323) -> ("session out"=w317:refnum<k21>, "error out"=w318:errorcluster)  [unwired: 12 in]
        n80 = call-poly <vilib>:"XNET Read.vi"("session in"=w317, "error in (no error)"=w318) -> ("session out"=w315:refnum<k21>, "data"=w308:dbl[], "error out"=w314:errorcluster)  [unwired: 11 in]
        n81 = property class="XNET Session"(reference=w315, error in=w314) -> (reference out=w312:refnum<k21>, error out=w313:errorcluster, "ListSigs"=w309:refnum<k21>[])
        n82 = call <vilib>:"XNET Clear.vi"("session in"=w312, "error in (no error)"=w313) -> ("error out"=w316:errorcluster)  [unwired: 13 in]
        n83 = for {
          tunnel: w309 -> [w328] mode=indexing
          tunnel: w308 -> [w327] mode=indexing
          tunnel: [w326] -> w307 mode=indexing
          n84 = Bundle By Name(cluster=T4 {"XNET Signal"="", "Data"=0.0} ("Signals OUT"), "XNET Signal"=w328, "Data"=w327) -> (w326:T4)
        }
      }
      frame "Read Frames Single" {
        n85 = for {
          tunnel: w344 -> [w356] mode=indexing
          tunnel: [w355] -> w343 mode=indexing
          n86 = Unbundle By Name(w356) -> ("Frame Name"=w355:refnum<k21>)
        }
        n87 = call-poly <vilib>:"XNET Create Session.vi"("frame list"=w343, "interface"=w332, "error in (no error)"=w341) -> ("session out"=w348:refnum<k21>, "error out"=w350:errorcluster)  [unwired: 11 in]
        n88 = property class="XNET Session"(reference=w348, error in=w350, "Intf.BaudRate64"=w335, "Intf.CAN.Term"=w334) -> (reference out=w347:refnum<k21>, error out=w349:errorcluster)
        n89 = call <vilib>:"XNET Start.vi"("session in"=w347, "error in (no error)"=w349) -> ("session out"=w346:refnum<k21>, "error out"=w345:errorcluster)  [unwired: 12 in]
        n90 = call-poly <vilib>:"XNET Read.vi"("session in"=w346, "error in (no error)"=w345) -> ("session out"=w338:refnum<k21>, "data"=w351:T2[], "error out"=w352:errorcluster)  [unwired: 10 in, 1 out]
        n91 = call "Convert Raw Frame to Data.vi"("Database alias"=w333, "error in (no error)"=w352, "Raw Frames"=w351) -> ("error out"=w340:errorcluster, "Frame Data"=w342:T1[])  [unwired: 7 in]
        n92 = call <vilib>:"XNET Clear.vi"("session in"=w338, "error in (no error)"=w340) -> ("error out"=w339:errorcluster)  [unwired: 13 in]
      }
      frame "Write Raw Frame Single" {
        n93 = for {
          tunnel: w364 -> [w379] mode=indexing
          tunnel: [w378] -> w358 mode=indexing
          n94 = Unbundle By Name(w379) -> ("Raw Frame"=w378:T2)
        }
        n95 = call "Convert Raw Frame to Data.vi"("Database alias"=w363, "error in (no error)"=w360, "Raw Frames"=w358) -> ("error out"=w361:errorcluster, "Frame Data"=w362:T1[])  [unwired: 7 in]
        n96 = for {
          tunnel: w362 -> [w377] mode=indexing
          tunnel: [w376] -> w359 mode=indexing
          n97 = Unbundle By Name(w377) -> ("Frame Name"=w376:refnum<k21>)
        }
        n98 = call-poly <vilib>:"XNET Create Session.vi"("frame list"=w359, "interface"=w357, "error in (no error)"=w361) -> ("session out"=w374:refnum<k21>, "error out"=w375:errorcluster)  [unwired: 11 in]
        n99 = call-poly <vilib>:"XNET Write.vi"("session in"=w374, "data"=w358, "error in (no error)"=w375) -> ("session out"=w371:refnum<k21>, "error out"=w372:errorcluster)  [unwired: 11 in]
        n100 = call <vilib>:"XNET Clear.vi"("session in"=w371, "error in (no error)"=w372) -> ("error out"=w370:errorcluster)  [unwired: 13 in]
      }
      frame "Write Raw Frame Session" {
        n101 = for {
          tunnel: w386 -> [w393] mode=indexing
          tunnel: [w392] -> w384 mode=indexing
          n102 = Unbundle By Name(w393) -> ("Raw Frame"=w392:T2)
        }
        n103 = call-poly <vilib>:"XNET Write.vi"("session in"=w382, "data"=w384, "error in (no error)"=w383) -> ("error out"=w381:errorcluster)  [unwired: 11 in, 1 out]
      }
      frame "FrameRef to Sigs" {
        n104 = Index Array(array=w401) -> (element=w395:T1)  [unwired: 1 in]
        n105 = Unbundle By Name(w395) -> ("Frame Name"=w394:refnum<k21>)
        n106 = property class="XNET Frame"(reference=w394, error in=w400) -> (error out=w397:errorcluster, "Sigs"=w399:refnum<k21>[])  [unwired: 1 out]
        n107 = for {
          tunnel: w399 -> [w410] mode=indexing
          tunnel: [w409] -> w398 mode=indexing
          n108 = Bundle By Name(cluster=T4 {"XNET Signal"="", "Data"=0.0} ("Signals OUT"), "XNET Signal"=w410) -> (w409:T4)
        }
      }
      frame "FrameID to FrameRef" {
        n109 = Index Array(array=w419) -> (element=w418:T1)  [unwired: 1 in]
        n110 = Unbundle By Name(w418) -> ("Raw Frame"=w417:T2)
        n111 = Unbundle By Name(w417) -> ("identifier"=w416:u32)
        n112 = call "FrameID to Frame Ref.vi"("Database alias"=w413, "error in (no error)"=w415, "Frame ID"=w416) -> ("error out"=w414:errorcluster)  [unwired: 6 in, 2 out]
      }
      frame "Close" {
        n113 = call <vilib>:"XNET Database Remove Alias.vi"("alias"=w426, "error in (no error)"=w440) -> ("error out"=w427:errorcluster)  [unwired: 13 in]
        n114 = call <vilib>:"XNET Clear.vi"("session in"=w436, "error in (no error)"=w427) -> ("error out"=w432:errorcluster)  [unwired: 13 in]
        n115 = call <vilib>:"XNET Clear.vi"("session in"=w435, "error in (no error)"=w427) -> ("error out"=w431:errorcluster)  [unwired: 13 in]
        n116 = call <vilib>:"XNET Clear.vi"("session in"=w434, "error in (no error)"=w427) -> ("error out"=w430:errorcluster)  [unwired: 13 in]
        n117 = call <vilib>:"XNET Clear.vi"("session in"=w433, "error in (no error)"=w427) -> ("error out"=w429:errorcluster)  [unwired: 13 in]
        n118 = Merge Errors(w432, w431, w430, w429) -> (w428:errorcluster)
        n119 = call <vilib>:"Clear Errors.vi"("error in (no error)"=w428) -> ()  [unwired: 5 in, 2 out]
      }
    }
  }
  "error out" <- w9
  "Signals OUT" <- w3
  "Frames OUT" <- w4
